vi "myRIO_BRig_RT_dataCurrent_Tcycle_generic.vi"() -> (2 "output_Tcycle_generic":i32)   [LabVIEW 2014]
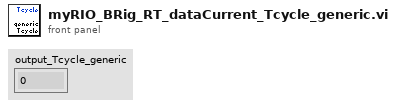
[diagram p1: front panel]
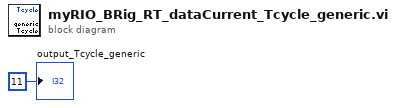
[diagram p0: block diagram]
diagram:
  "output_Tcycle_generic" <- 11 ("output_iBlock")
